vi "Translator.Global.vi"() -> ()   [LabVIEW 2016]
panel:
  in  "TranslatedVIs 2":string[](array[string])=["MainGui.vi", "Translator.MainGui.vi", "Translator.SelectLanguageGui.vi", "User.LoginGui.vi", "User.SettingsGui.vi", "EventLog.Gui.vi", "ErrorHandling.Gui.vi", "Wait.Gui.vi", "AboutGui.vi", "InfoGui.vi", "ExitGui.vi", "Station.Gui.vi:1", "Station.Gui.vi:2", "Station.Gui.vi:3", "Station.Gui.vi:4", "Station.Gui.vi:5", "Station.Gui.vi:6"]
  in  "tab":enum32{"General", "Daq"}(tab)
  out "Translations.TimeSpan":string[](array[string])
  out "Translations.ResOptions":string[](array[string])
  out "Translations.GuiMode":string[](array[string])
  out "Translations.TestStatus":string[](array[string])
  out "Translations.Months":string[](array[string])
  out "Translations.Source":string[](array[string])
  out "Translations.Msg":string[](array[string])
  out "Translations.Level":string[](array[string])
  out "Translations.ExitAction":string[](array[string])
  out "Translations.Daq.Msg":string[](array[string])
  out "Translations.Daq.CNT":string[](array[string])
  out "Translations.Daq.AO":string[](array[string])
  out "Translations.Daq.AI":string[](array[string])
  out "Translations.Daq.DI":string[](array[string])
  out "Translations.Daq.DO":string[](array[string])
  in  "FilePath":path
  out "Font":string
  in  "TranslatedVIs":string[](array[string])
  in  "Applicaiton INI file":path
  out "Languages":string[](array[string])
  out "Flag":picture
  # "-> not used anymore; VIs translated separately inside its VI"
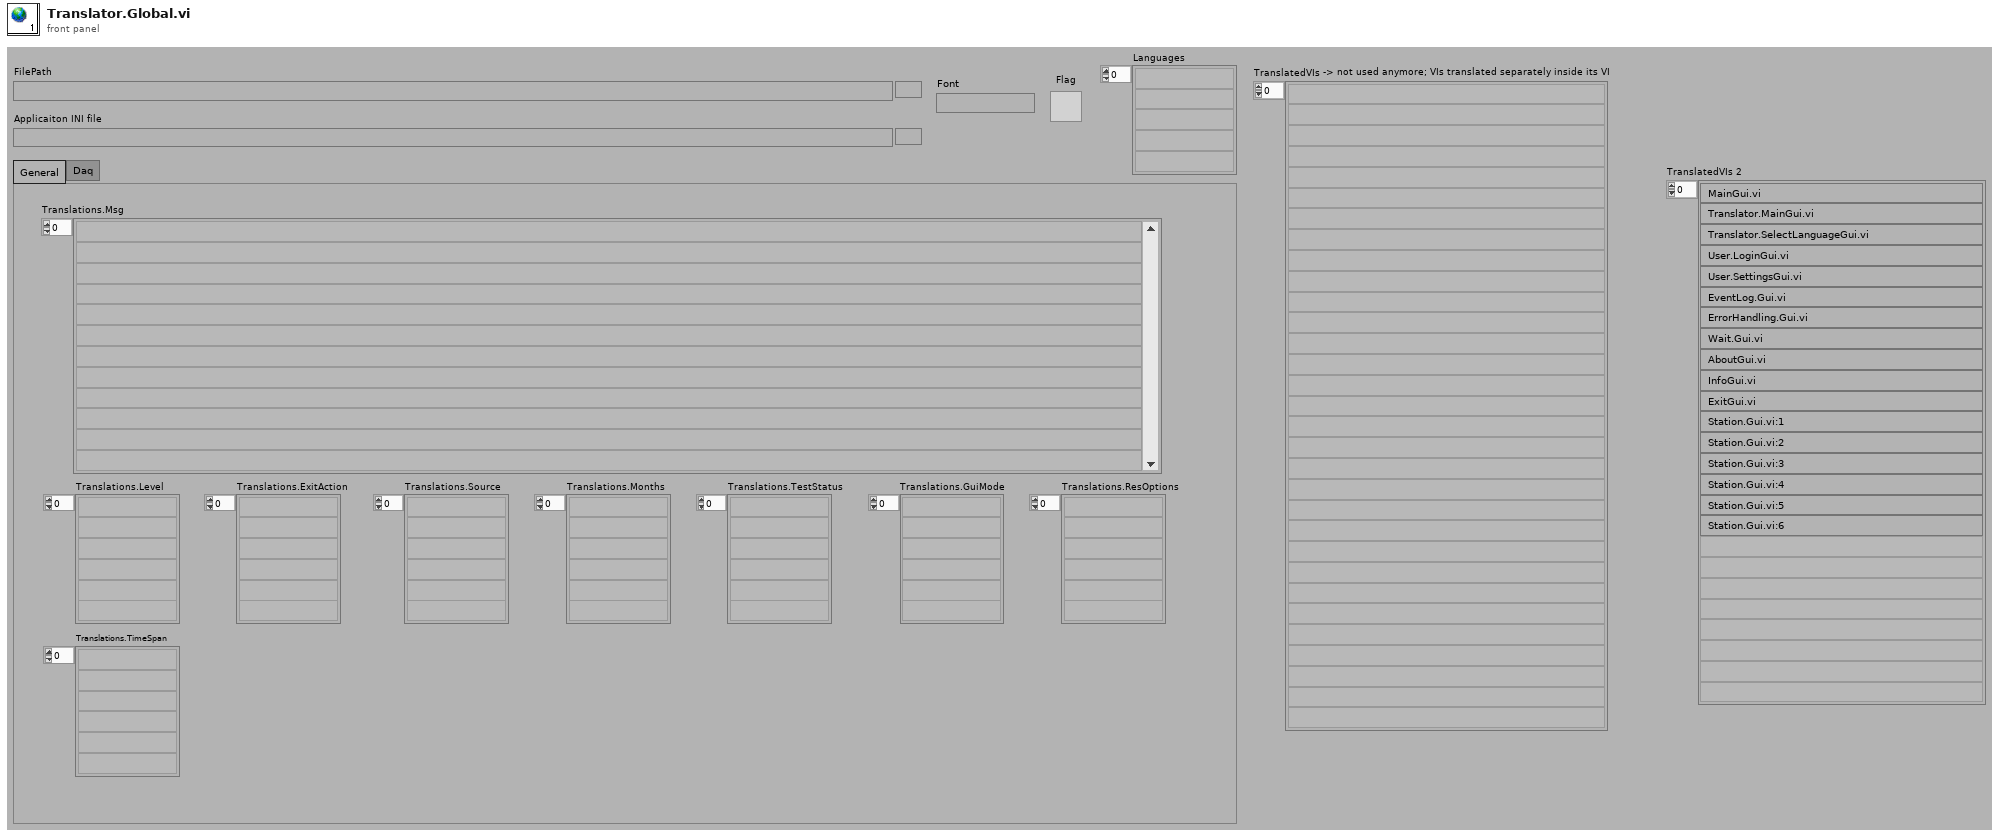
[diagram p1: front panel]
diagram:
